vi "SetParam.vi"(8 "error in (no error)":errorcluster caption="entrée d'erreur (pas d'erreur)", 10 "SimpleImputer":T1={"missing_values"="nan", "strategy"="mean", "fill_value"={"dtype"="", "str"="None", "int"=0}, "verbose"=0, "copy"=TRUE, "add_indicator"=FALSE}, 11 "SimpleImputer.lvclass":refnum<class "SimpleImputer.lvclass">) -> (0 "error out":errorcluster caption="sortie d'erreur", 3 "SimpleImputer.lvclass":refnum<class "SimpleImputer.lvclass">)   [LabVIEW 2020, in "SimpleImputer.lvclass"]
doc: "Set Parameters"
uses:
  SimpleImputer.lvclass
  SimpleImputer.lvclass/SimpleImputer.ctl
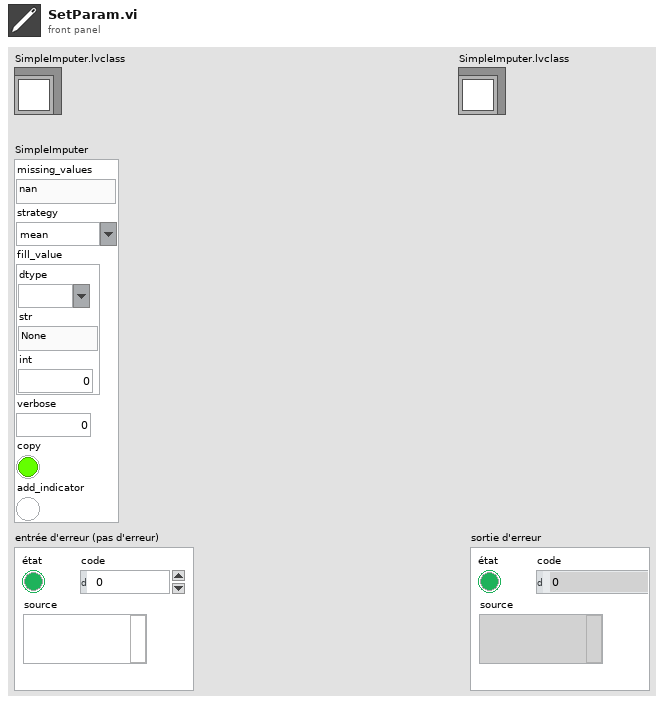
[diagram p1: front panel]
types:
  T1 = cluster{"missing_values":string, "strategy":string, "fill_value":cluster{"dtype":string, "str":string, "int":i32}, "verbose":i32, "copy":bool, "add_indicator":bool}
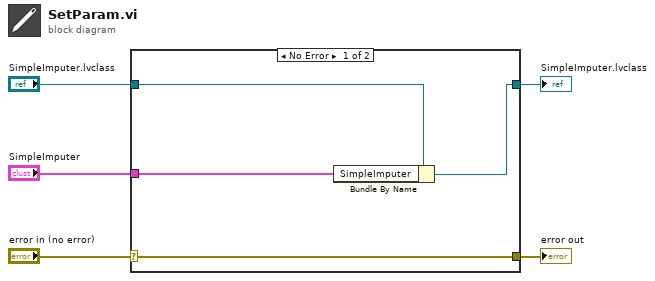
[diagram p0: block diagram]
diagram:
  n1 = case shown="No Error" "error in (no error)" {
    selector: "error in (no error)" -> [w9 w10]
    tunnel: [w9 w10] -> w4
    tunnel: [w7 w11] -> w2
    tunnel: "SimpleImputer.lvclass" -> [w8 w11]
    tunnel: "SimpleImputer" -> [w6 _]
    frame No Error {
      n2 = Bundle By Name(cluster=w8, "SimpleImputer"=w6) -> (w7:refnum<class "SimpleImputer.lvclass">)
    }
    frame Error {
    }
  }
  "error out" <- w4
  "SimpleImputer.lvclass" <- w2
